vi "io_parse_bin_data_header.vi"(7 "Error when unrecognised header (T)":bool=TRUE, 8 "error in":errorcluster, 11 "VISA resource name":refnum<visa-resource-name>) -> (0 "error out":errorcluster, 1 "First character out":string, 2 "Size of the bin data":i64, 3 "VISA resource name out":refnum<visa-resource-name>)   [LabVIEW 2014, in "rszvl_rsidr_core.lvlib"]
uses:
  rszvl_rsidr_core.lvlib
  type_Error_Codes.ctl
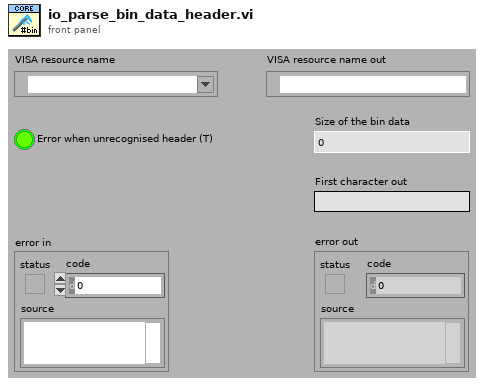
[diagram p1: front panel]
types:
  T1 = typedef "rszvl_rsidr_core.lvlib/type_Session_Data.ctl" = cluster{"Instr type":string, "Instr type for err. msg.":string, "Installed Options":string[], "OPC Timeout":i32, "Query Instrument Status":bool, "Check Range":bool, "Check Options":bool, "Add LF to Write":bool, "Simulate":bool, "Logging":bool, "Logging params":variant, "Interface Type":enum16{"Unknown", "GPIB", "VXI", "GPIB_VXI", "ASRL", "PXI", "TCPIP", "USB", "SOCKET"}, "Fast Sweep":i32, "AdditionalFlags":i32, "WaitBeforeWrite":i32, "WaitBeforeRead":i32, "BinDataChunkSize":i64}
  T2 = typedef "rszvl_rsidr_core.lvlib/type_Error_Codes.ctl" = enum16{"No_error", "VISA_err_ResourceNotFound", "VISA_err_Timeout", "VISA_warn_MoreDataAvailable", "RS_err_MissingCallback", "RS_err_InvalidAttribute", "RS_err_InvalidValue", "RS_err_UnknownResource", "RS_err_AlreadyInitialized", "RS_err_InstrumentStatus", "RS_err_BadRepCapName", "RS_err_TypesMismatch", "RS_err_ValueNotSupported", "RS_err_InvalidRngTable", "RS_err_IDqueryFail", "RS_err_UnexpResponse", "VISA_warn_ConfigNotLoaded", "RS_err_AttributeNotReadable", "RS_err_AttributeNotWritable", "RS_err_InstrumentType", "RS_err_InstrumentOption", "VISA_err_InvalidSize", "RS_err_ReliabilityIndicator", "VISA_warn_UnknownStatus", "VISA_warn_TermCharRead", "VISA_err_IO_error"}
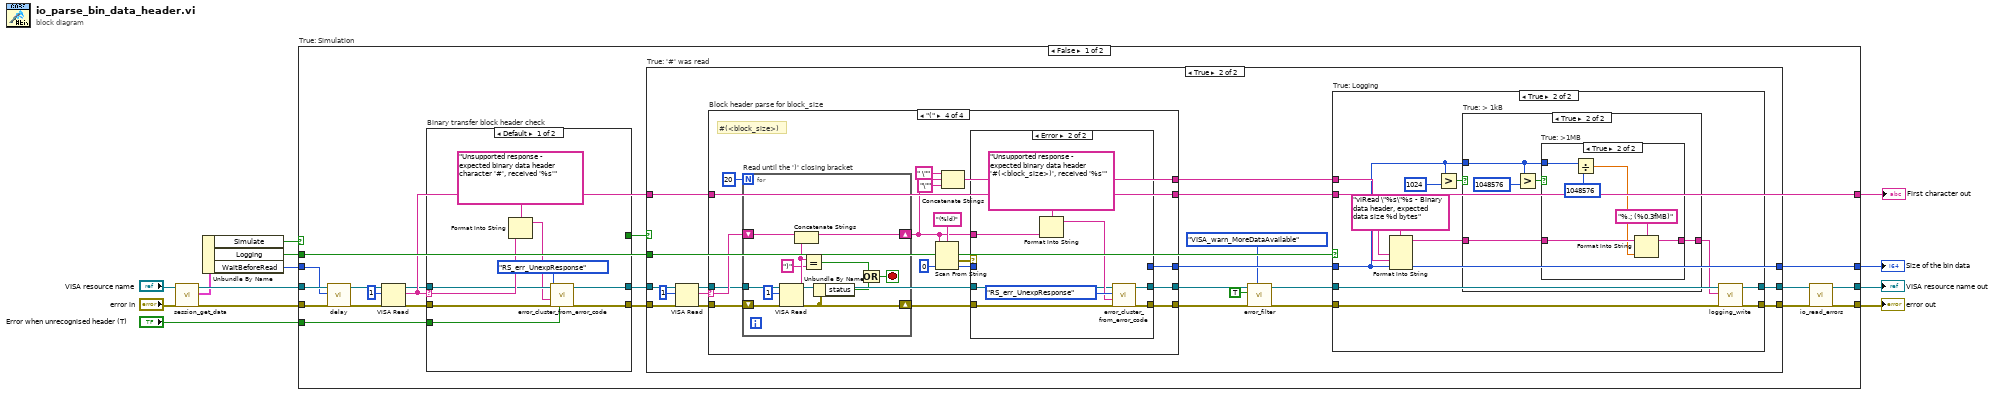
[diagram p0: block diagram]
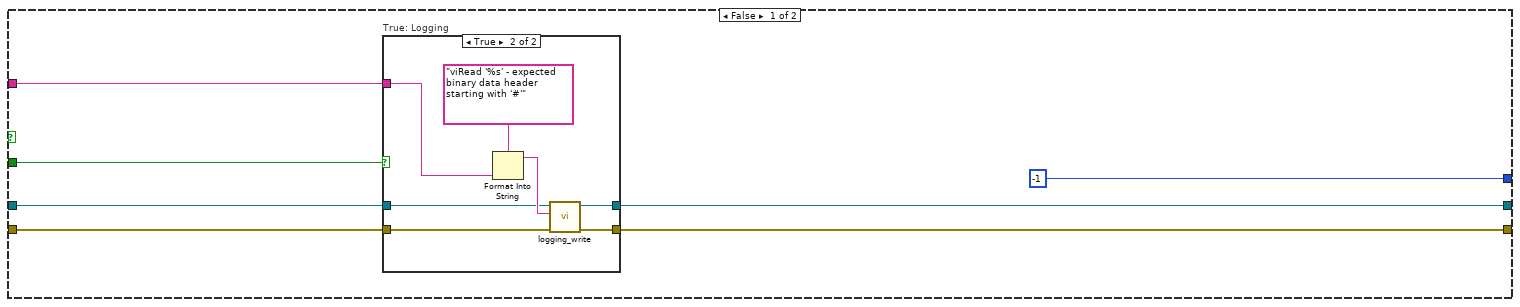
[diagram p2: hidden frame]
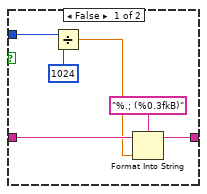
[diagram p6: hidden frame]
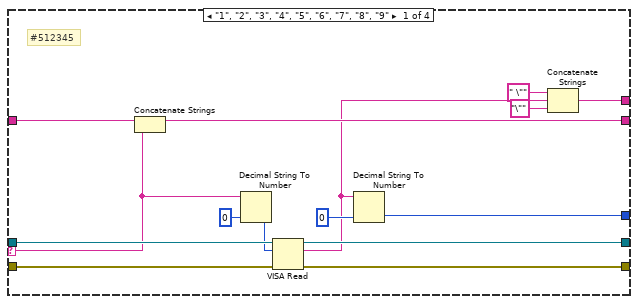
[diagram p7: hidden frame]
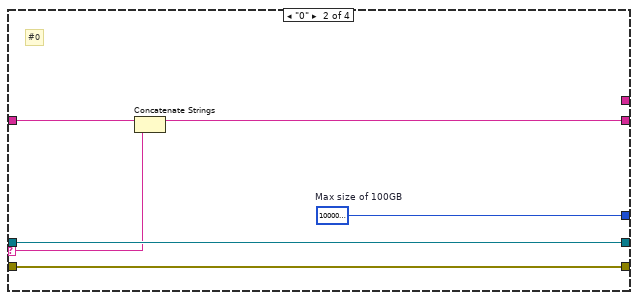
[diagram p8: hidden frame]
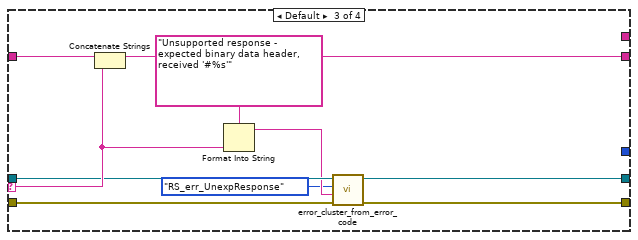
[diagram p9: hidden frame]
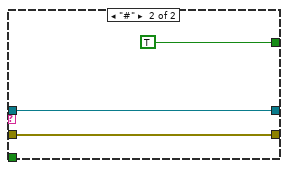
[diagram p11: hidden frame]
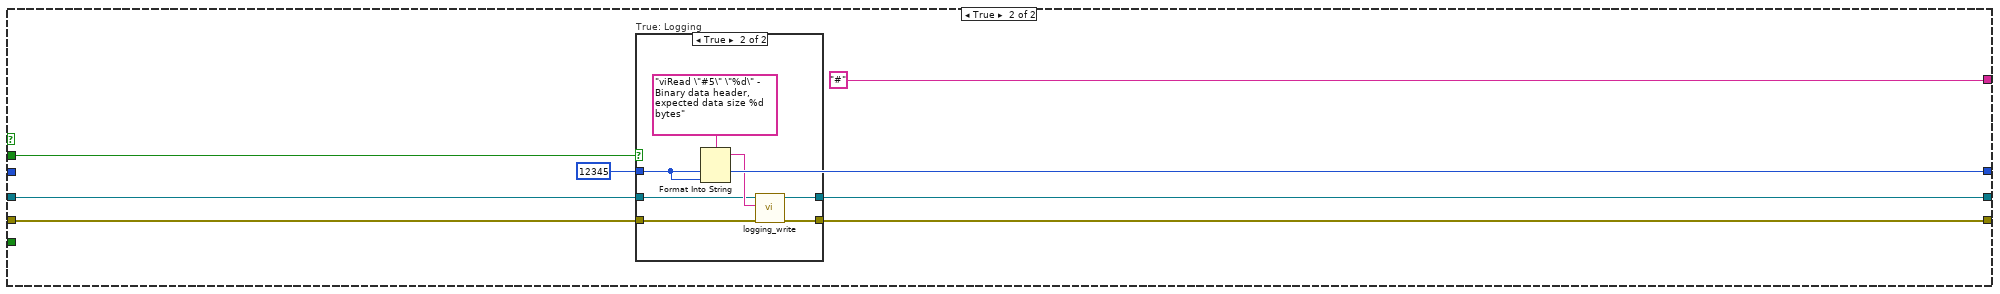
[diagram p12: hidden frame]
diagram:
  n1 = call "session_get_data.vi"("error in"="error in", "VISA resource name"="VISA resource name") -> ("error out"=w8:errorcluster, "Session User Data out"=w5:T1, "VISA resource name out"=w7:refnum<visa-resource-name>)  [unwired: 7 in]
  n2 = Unbundle By Name(w5) -> ("Simulate"=w6:bool, "Logging"=w4:bool, "WaitBeforeRead"=w1:i32)
  n3 = case "True: Simulation" shown="False" w6 {
    tunnel: [w28 w188] -> w13
    tunnel: w8 -> [w18 w187]
    tunnel: w7 -> [w17 w186]
    tunnel: [w20 w185] -> w12
    tunnel: [w19 w184] -> w11
    tunnel: w4 -> [w29 w183]
    tunnel: "Error when unrecognised header (T)" -> [w27 _]
    tunnel: [w25 "#" ("read buffer")] -> w2
    tunnel: w1 -> [w14 _]
    frame False {
      n4 = call "delay.vi"("error in"=w18, "Milliseconds to wait"=w14, "VISA resource name"=w17) -> ("error out"=w16:errorcluster, "VISA resource name out"=w15:refnum<visa-resource-name>)  [unwired: 7 in]
      n5 = VISA Read(VISA resource name=w15, byte count=u32 1 ("byte count (0)"), error in (no error)=w16) -> (VISA resource name out=w24:refnum<visa-resource-name>, read buffer=w25:string, error out=w31:errorcluster)  [unwired: 1 out]
      n6 = case "Binary transfer block header check" shown="Default" w25 {
        selector: w25 -> [w177 _]
        tunnel: w31 -> [w176 w181]
        tunnel: [w175 w181] -> w30
        tunnel: w27 -> [w174 _]
        tunnel: [_ TRUE ("Error when unrecognised header (T)")] -> w26
        tunnel: w24 -> [w173 w179]
        tunnel: [w170 w179] -> w23
        frame Default {
          n7 = Format Into String(format string="Unsupported response - expected binary data header character '#', received '%s'" ("error message (\"\")"), w177) -> (resulting string=w171:string)  [unwired: 2 in, 1 out]
          n8 = call "error_cluster_from_error_code.vi"("error creation enabled (T)"=w174, "error in"=w176, "error message (\"\")"=w171, "Error Enum in"=type_Error_Codes."RS_err_UnexpResponse", "VISA resource name"=w173) -> ("error out"=w175:errorcluster, "VISA resource name out"=w170:refnum<visa-resource-name>)  [unwired: 5 in]
        }
        frame "#" {
        }
      }
      n9 = case "True: '#' was read" shown="True" w26 {
        tunnel: w30 -> [w38 w66]
        tunnel: w23 -> [w37 w62]
        tunnel: [w36 w61] -> w22
        tunnel: [w35 w60] -> w21
        tunnel: w29 -> [w34 w59]
        tunnel: w25 -> [w33 w58]
        tunnel: [i64 -1 ("default value 1") w55] -> w28
        frame False {
          n10 = case "True: Logging" shown="True" w34 {
            tunnel: w38 -> [w40 w46]
            tunnel: w37 -> [w41 w45]
            tunnel: [w40 w44] -> w36
            tunnel: [w41 w43] -> w35
            tunnel: w33 -> [_ w42]
            frame False {
            }
            frame True {
              n11 = Format Into String(format string="viRead '%s' - expected binary data header starting with '#'" ("String to write"), w42) -> (resulting string=w47:string)  [unwired: 2 in, 1 out]
              n12 = call "logging_write.vi"("error in"=w46, "String to write"=w47, "VISA resource name"=w45) -> ("error out"=w44:errorcluster, "VISA resource name out"=w43:refnum<visa-resource-name>)  [unwired: 7 in]
            }
          }
        }
        frame True {
          n13 = VISA Read(VISA resource name=w62, byte count=u32 1 ("byte count (0)"), error in (no error)=w66) -> (VISA resource name out=w63:refnum<visa-resource-name>, read buffer=w64:string, error out=w65:errorcluster)  [unwired: 1 out]
          n14 = case "Block header parse for block_size" shown="\"(\"" w64 {
            selector: w64 -> [w104 w117 w127 w146]
            tunnel: w65 -> [w114 w120 w126 w147]
            tunnel: w63 -> [w113 w119 w125 w132]
            tunnel: [w111 w115 _ w138] -> w55
            tunnel: [w109 w120 w124 w140] -> w54
            tunnel: [w108 w119 w123 w131] -> w50
            tunnel: w58 -> [w106 w118 w128 w137]
            tunnel: [w105 w116 w129 w137] -> w57
            tunnel: [w103 _ _ w134] -> w56
            frame "1", "2", "3", "4", "5", "6", "7", "8", "9" {
              # "#512345"
              n15 = Concatenate Strings(w106, w104) -> (w105:string)
              n16 = Decimal String To Number(string=w104, default (0L)=u32 0 ("default (0 I32)")) -> (number=w112:u32)  [unwired: 1 in, 1 out]
              n17 = VISA Read(VISA resource name=w113, byte count=w112, error in (no error)=w114) -> (VISA resource name out=w108:refnum<visa-resource-name>, read buffer=w102:string, error out=w109:errorcluster)  [unwired: 1 out]
              n18 = Decimal String To Number(string=w102, default (0L)=i64 0 ("default (0 I32)")) -> (number=w111:i64)  [unwired: 1 in, 1 out]
              n19 = Concatenate Strings(" \"" ("string"), w102, "\"" ("string")) -> (w103:string)
            }
            frame "0" {
              w115 = i64 100000000000  # Max size of 100GB
              # "#0"
              n20 = Concatenate Strings(w118, w117) -> (w116:string)
            }
            frame Default {
              n21 = Concatenate Strings(w128, w127) -> (w129:string)
              n22 = Format Into String(format string="Unsupported response - expected binary data header, received '#%s'" ("error message (\"\")"), w127) -> (resulting string=w122:string)  [unwired: 2 in, 1 out]
              n23 = call "error_cluster_from_error_code.vi"("error in"=w126, "error message (\"\")"=w122, "Error Enum in"=type_Error_Codes."RS_err_UnexpResponse", "VISA resource name"=w125) -> ("error out"=w124:errorcluster, "VISA resource name out"=w123:refnum<visa-resource-name>)  [unwired: 6 in]
            }
            frame "(" {
              # "#(<block_size>)"
              n24 = for "Read until the ')' closing bracket" {
                N: 20 -> [_]
                tunnel: w132 -> [w158]
                shift-right: [w155] -> w136
                shift-left: w146 -> [w156]
                shift-right: [w152] -> w142
                shift-left: w147 -> [w157]
                stop <- w149 stop-if-true
                n25 = VISA Read(VISA resource name=w158, byte count=u32 1, error in (no error)=w157) -> (read buffer=w154:string, error out=w152:errorcluster)  [unwired: 2 out]
                n26 = Concatenate Strings(w156, w154) -> (w155:string)
                n27 = Equal?(x=w154, y=")") -> (x = y?=w150:bool)
                n28 = Unbundle By Name(w152) -> ("status"=w151:bool)
                n29 = Or(x=w150, y=w151) -> (x .or. y?=w149:bool)
              }
              n30 = Scan From String(format string="(%ld)", input string=w136, default 1=i64 0 ("default value 1")) -> (error out=w143:errorcluster, output 1=w139:i64)  [unwired: 2 in, 2 out]
              n31 = Concatenate Strings(" \"" ("string"), w136, "\"" ("string")) -> (w134:string)
              n32 = case shown="Error" w143 {
                tunnel: w142 -> [w160 w166]
                tunnel: w136 -> [_ w168]
                tunnel: [w160 w167] -> w140
                tunnel: w139 -> [w161 _]
                tunnel: [w161 _] -> w138
                tunnel: w132 -> [w159 w163]
                tunnel: [w159 w162] -> w131
                frame No Error {
                }
                frame Error {
                  n33 = Format Into String(format string="Unsupported response - expected binary data header  '#(<block_size>)', received '%s'" ("error message (\"\")"), w168) -> (resulting string=w164:string)  [unwired: 2 in, 1 out]
                  n34 = call "error_cluster_from_error_code.vi"("error in"=w166, "error message (\"\")"=w164, "Error Enum in"=type_Error_Codes."RS_err_UnexpResponse", "VISA resource name"=w163) -> ("error out"=w167:errorcluster, "VISA resource name out"=w162:refnum<visa-resource-name>)  [unwired: 6 in]
                }
              }
            }
          }
          n35 = call "error_filter.vi"("Error Enum in"=type_Error_Codes."VISA_warn_MoreDataAvailable", "error in"=w54, "Clear detected code (F)"=TRUE, "VISA resource name"=w50) -> ("error out"=w53:errorcluster, "VISA resource name out"=w49:refnum<visa-resource-name>)  [unwired: 5 in, 1 out]
          n36 = case "True: Logging" shown="True" w59 {
            tunnel: w53 -> [w68 w81]
            tunnel: w49 -> [w69 w80]
            tunnel: [w68 w79] -> w61
            tunnel: [w69 w78] -> w60
            tunnel: w57 -> [_ w76]
            tunnel: w56 -> [_ w75]
            tunnel: w55 -> [_ w72]
            frame False {
            }
            frame True {
              n37 = Format Into String(format string="viRead \"%s\"%s - Binary data header, expected data size %d bytes" ("String to write"), w76, w75, w72) -> (resulting string=w71:string)  [unwired: 2 in, 1 out]
              n38 = Greater?(x=w72, y=i64 1024) -> (0:w73:bool)
              n39 = case "True: > 1kB" shown="True" w73 {
                tunnel: w72 -> [_ w85]
                tunnel: w71 -> [w82 w84]
                tunnel: [w82 w83] -> w70
                frame False {
                }
                frame True {
                  n40 = Greater?(x=w85, y=i64 1048576) -> (0:w86:bool)
                  n41 = case "True: >1MB" shown="True" w86 {
                    tunnel: w85 -> [w90 w96]
                    tunnel: w84 -> [w92 w98]
                    tunnel: [w91 w97] -> w83
                    frame False {
                      n42 = Divide(x=w90, y=i64 1024) -> (x/y=w88:dbl)
                      n43 = Format Into String(format string="%.; (%0.3fkB)", initial string=w92, w88) -> (resulting string=w91:string)  [unwired: 1 in, 1 out]
                    }
                    frame True {
                      n44 = Divide(x=w96, y=i64 1048576) -> (x/y=w95:dbl)
                      n45 = Format Into String(format string="%.; (%0.3fMB)", initial string=w98, w95) -> (resulting string=w97:string)  [unwired: 1 in, 1 out]
                    }
                  }
                }
              }
              n46 = call "logging_write.vi"("error in"=w81, "String to write"=w70, "VISA resource name"=w80) -> ("error out"=w79:errorcluster, "VISA resource name out"=w78:refnum<visa-resource-name>)  [unwired: 7 in]
            }
          }
        }
      }
      n47 = call "io_read_errors.vi"("error in"=w22, "VISA resource name"=w21) -> ("error out"=w20:errorcluster, "VISA resource name out"=w19:refnum<visa-resource-name>)  [unwired: 8 in]
    }
    frame True {
      w188 = i64 12345 ("default value 1")
      n48 = case "True: Logging" shown="True" w183 {
        tunnel: w187 -> [w189 w195]
        tunnel: w186 -> [w190 w194]
        tunnel: [w189 w193] -> w185
        tunnel: [w190 w192] -> w184
        tunnel: w188 -> [_ w191]
        frame False {
        }
        frame True {
          n49 = Format Into String(format string="viRead \"#5\" \"%d\" - Binary data header, expected data size %d bytes" ("String to write"), w191, w191) -> (resulting string=w196:string)  [unwired: 2 in, 1 out]
          n50 = call "logging_write.vi"("error in"=w195, "String to write"=w196, "VISA resource name"=w194) -> ("error out"=w193:errorcluster, "VISA resource name out"=w192:refnum<visa-resource-name>)  [unwired: 7 in]
        }
      }
    }
  }
  "error out" <- w12
  "VISA resource name out" <- w11
  "Size of the bin data" <- w13
  "First character out" <- w2
